vi "m2aadtView.vi"   [LabVIEW 2013, in "M2AADTViews.lvlib"]
uses:
  M2AADTViews.lvlib
  CommandFactory/CommandFactory.lvclass
  UserEvents/UserEvents.lvclass
  UserEvents/UserEvents.lvclass/UserEvents.ctl
  Typedefs/CommandSelector.ctl
  Typedefs/StateSelector.ctl
  Typedefs/M2AADTTypedefs.lvlib
  Controller/Controller.lvclass
  ConfigurationThisComponent/ConfigurationThisComponent.lvclass
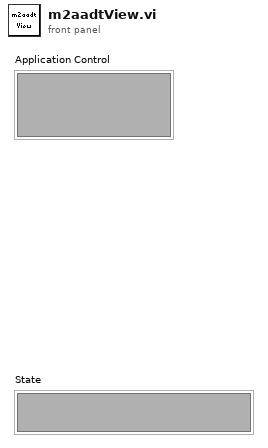
[diagram p1: front panel]
types:
  T1 = enum32{"invalid app kind", "Development System", "Run Time System", "Student Edition", "Embedded LabVIEW", "Evaluation", "Custom"}
  T2 = typedef "M2AADTTypedefs.lvlib/PubDataEvents.ctl" = cluster{"State":refnum<user-event>, "ErrorCode":refnum<user-event>, "OutputData":refnum<user-event>, "InputData":refnum<user-event>, "ControllerData":refnum<user-event>, "TestStatus":refnum<user-event>, "LogPath":refnum<user-event>, "StiffnessData":refnum<user-event>}
  T3 = typedef "M2AADTTypedefs.lvlib/SubDataEvents.ctl" = cluster{"Command":refnum<user-event>}
  T4 = cluster{"Event Registration Refnum":refnum<event-registration>, "Event Registration Refnum":refnum<event-registration>}
  T5 = typedef "M2AADTTypedefs.lvlib/CommandSelector.ctl" = enum16{"ClearError", "EnableMotion", "Exit", "ForceDemand", "StandBy", "Start", "StartAutomatedTest", "StopAutomatedTest", "StopMotion", "Update"}
  T6 = typedef "M2AADTTypedefs.lvlib/StateSelector.ctl" = enum16{"EndingCycleState", "FaultState", "InteractiveMotionState", "MovingToNewForceState", "OffState", "PausingState", "StandbyState", "StoppedState"}
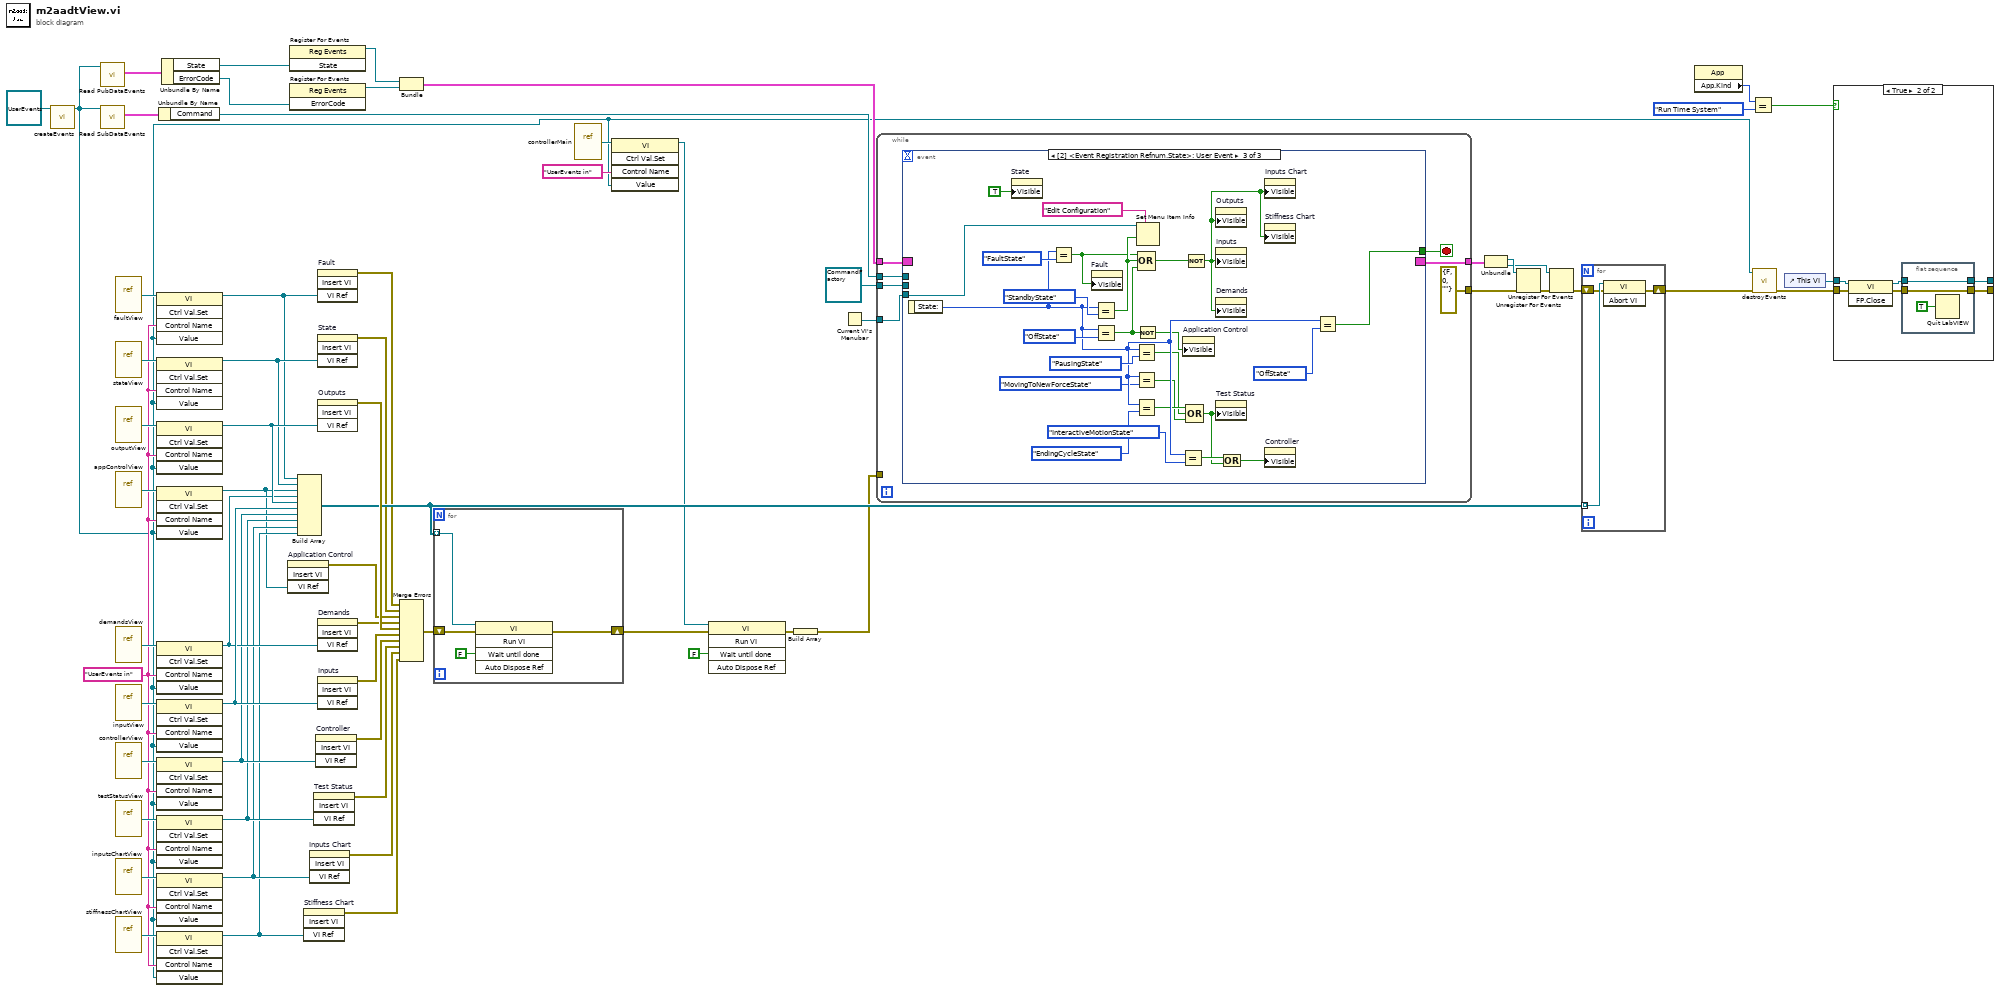
[diagram p0: block diagram]
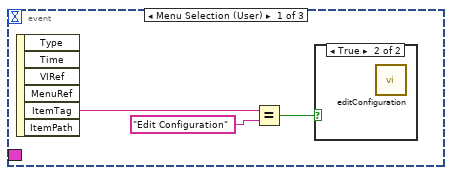
[diagram p3: hidden frame]
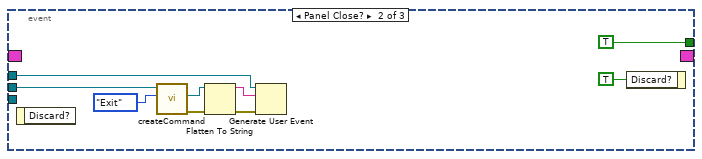
[diagram p5: hidden frame]
diagram:
  w6 = "UserEvents in" ("Control Name")
  n1 = call "createEvents.vi"("UserEvents in"=refnum<class "UserEvents.lvclass"> refnum) -> ("UserEvents out"=w5:refnum<class "UserEvents.lvclass">)  [unwired: 9 in, 1 out]
  n2 = call "Read PubDataEvents.vi"("UserEvents in"=w5) -> ("PubDataEvents"=w55:T2)  [unwired: 9 in, 1 out]
  n3 = call "Read SubDataEvents.vi"("UserEvents in"=w5) -> ("SubDataEvents"=w53:T3)  [unwired: 9 in, 1 out]
  n4 = vi-ref "faultView.vi"() -> (w7:refnum<vi>)
  n5 = vi-ref "stateView.vi"() -> (w10:refnum<vi>)
  n6 = vi-ref "outputView.vi"() -> (w35:refnum<vi>)
  n7 = vi-ref "appControlView.vi"() -> (w14:refnum<vi>)
  n8 = vi-ref "demandsView.vi"() -> (w29:refnum<vi>)
  n9 = vi-ref "inputView.vi"() -> (w43:refnum<vi>)
  n10 = vi-ref "controllerView.vi"() -> (w26:refnum<vi>)
  n11 = vi-ref "testStatusView.vi"() -> (w25:refnum<vi>)
  n12 = vi-ref "inputsChartView.vi"() -> (w20:refnum<vi>)
  n13 = vi-ref "stiffnessChartView.vi"() -> (w17:refnum<vi>)
  n14 = invoke class="VI" method="Ctrl Val.Set"(reference=w7, "Control Name"=w6, "Value"=w5) -> (reference out=w4:refnum<vi>)  [unwired: 2 in, 4 out]
  n15 = invoke class="VI" method="Ctrl Val.Set"(reference=w10, "Control Name"=w6, "Value"=w5) -> (reference out=w9:refnum<vi>)  [unwired: 2 in, 4 out]
  n16 = invoke class="VI" method="Ctrl Val.Set"(reference=w35, "Control Name"=w6, "Value"=w5) -> (reference out=w34:refnum<vi>)  [unwired: 2 in, 4 out]
  n17 = invoke class="VI" method="Ctrl Val.Set"(reference=w14, "Control Name"=w6, "Value"=w5) -> (reference out=w12:refnum<vi>)  [unwired: 2 in, 4 out]
  n18 = invoke class="VI" method="Ctrl Val.Set"(reference=w29, "Control Name"=w6, "Value"=w5) -> (reference out=w28:refnum<vi>)  [unwired: 2 in, 4 out]
  n19 = invoke class="VI" method="Ctrl Val.Set"(reference=w43, "Control Name"=w6, "Value"=w5) -> (reference out=w33:refnum<vi>)  [unwired: 2 in, 4 out]
  n20 = invoke class="VI" method="Ctrl Val.Set"(reference=w26, "Control Name"=w6, "Value"=w5) -> (reference out=w24:refnum<vi>)  [unwired: 2 in, 4 out]
  n21 = invoke class="VI" method="Ctrl Val.Set"(reference=w25, "Control Name"=w6, "Value"=w5) -> (reference out=w23:refnum<vi>)  [unwired: 2 in, 4 out]
  n22 = invoke class="VI" method="Ctrl Val.Set"(reference=w20, "Control Name"=w6, "Value"=w5) -> (reference out=w18:refnum<vi>)  [unwired: 2 in, 4 out]
  n23 = invoke class="VI" method="Ctrl Val.Set"(reference=w17, "Control Name"=w6, "Value"=w5) -> (reference out=w16:refnum<vi>)  [unwired: 2 in, 4 out]
  n24 = Unbundle By Name(w53) -> ("Command"=w52:refnum<user-event>)
  n25 = Unbundle By Name(w55) -> ("State"=w51:refnum<user-event>, "ErrorCode"=w49:refnum<user-event>)
  n26 = invoke on="Application Control" class="SubPnl" method="Insert VI"("VI Ref"=w12) -> (error out=w13:errorcluster)  [unwired: 3 in, 3 out]
  n27 = register-events(w51) -> (reference out=w50:refnum<event-registration>)  [unwired: 2 in, 1 out]
  n28 = register-events(w49) -> (reference out=w48:refnum<event-registration>)  [unwired: 2 in, 1 out]
  n29 = Build Array(w4, w9, w12, w28, w34, w33, w24, w23, w18, w16) -> (w58:refnum<vi>[])
  n30 = invoke on="Stiffness Chart" class="SubPnl" method="Insert VI"("VI Ref"=w16) -> (error out=w15:errorcluster)  [unwired: 3 in, 3 out]
  n31 = invoke on="Inputs Chart" class="SubPnl" method="Insert VI"("VI Ref"=w18) -> (error out=w19:errorcluster)  [unwired: 3 in, 3 out]
  n32 = invoke on="Test Status" class="SubPnl" method="Insert VI"("VI Ref"=w23) -> (error out=w21:errorcluster)  [unwired: 3 in, 3 out]
  n33 = invoke on="Controller" class="SubPnl" method="Insert VI"("VI Ref"=w24) -> (error out=w22:errorcluster)  [unwired: 3 in, 3 out]
  n34 = invoke on="Fault" class="SubPnl" method="Insert VI"("VI Ref"=w4) -> (error out=w3:errorcluster)  [unwired: 3 in, 3 out]
  n35 = invoke on="State" class="SubPnl" method="Insert VI"("VI Ref"=w9) -> (error out=w8:errorcluster)  [unwired: 3 in, 3 out]
  n36 = invoke on="Outputs" class="SubPanel" method="Insert VI"("VI Ref"=w34) -> (error out=w61:errorcluster)  [unwired: 3 in, 3 out]
  n37 = invoke on="Demands" class="SubPanel" method="Insert VI"("VI Ref"=w28) -> (error out=w27:errorcluster)  [unwired: 3 in, 3 out]
  n38 = invoke on="Inputs" class="SubPnl" method="Insert VI"("VI Ref"=w33) -> (error out=w60:errorcluster)  [unwired: 3 in, 3 out]
  n39 = Bundle("Event Registration Refnum"=w50, "Event Registration Refnum"=w48) -> (w41:T4)  [unwired: 1 in]
  n40 = Merge Errors(w3, w8, w13, w27, w61, w60, w22, w21, w19, w15) -> (w59:errorcluster)
  n41 = for {
    tunnel: w58 -> [w68] mode=indexing
    shift-right: [w67] -> w11
    shift-left: w59 -> [w66]
    n42 = invoke class="VI" method="Run VI"(reference=w68, error in=w66, "Wait until done"=FALSE ("Wait Until Done")) -> (error out=w67:errorcluster)  [unwired: 2 in, 4 out]
  }
  n43 = vi-ref "controllerMain.vi"() -> (w46:refnum<vi>)
  n44 = invoke class="VI" method="Ctrl Val.Set"(reference=w46, "Control Name"="UserEvents in", "Value"=w5) -> (reference out=w44:refnum<vi>)  [unwired: 2 in, 4 out]
  n45 = invoke class="VI" method="Run VI"(reference=w44, error in=w11, "Wait until done"=FALSE ("Wait Until Done")) -> (error out=w30:errorcluster)  [unwired: 2 in, 4 out]
  n46 = Build Array(w30) -> (w31:errorcluster[])
  n47 = Current VI's Menubar() -> (w56:refnum<k9>)
  n48 = while {
    tunnel: refnum<class "CommandFactory.lvclass"> refnum ("CommandFactory.lvclass") -> [w72]
    tunnel: [errorcluster {"status"=FALSE, "code"=0, "source"=""} ("error out")] -> w42
    tunnel: w56 -> [w70]
    tunnel: w41 -> [w74]
    tunnel: w52 -> [w71]
    tunnel: [w69] -> w40
    tunnel: w31 -> [_]
    stop <- w73 stop-if-true
    n49 = event shown="[2] <Event Registration Refnum.State>: User Event" {
      selector: w74 -> [_ _ _]
      dyn-events: [_ _ _] -> w69
      timeout: _ -> [_ _ _]
      tunnel: [_ TRUE w106] -> w73
      tunnel: w72 -> [_ w82 _]
      tunnel: w71 -> [_ w79 _]
      tunnel: w70 -> [_ _ w108]
      event Menu Selection (User) {
        n50 = event-data() -> ("ItemTag"=w76:string)  [unwired: 1 in, 5 out]
        n51 = Equal?(x=w76, y="Edit Configuration") -> (x = y?=w78:bool)
        n52 = case shown="True" w78 {
          frame False {
          }
          frame True {
            n53 = call "editConfiguration.vi"() -> ()  [unwired: 10 in, 2 out]
          }
        }
      }
      event Panel Close? {
        n54 = event-data() -> ()  [unwired: 1 in, 1 out]
        n55 = call-dynamic "createCommand.vi"("Command"=CommandSelector."Exit", "CommandFactory in"=w82) -> ("error out"=w87:errorcluster, "command"=w86:refnum<class "Command.lvclass">)  [unwired: 7 in, 1 out]
        n56 = Flatten To String(anything=w86, error in (no error)=w87) -> (data string=w80:string, error out=w81:errorcluster)  [unwired: 2 in, 1 out]
        n57 = Generate User Event(user event=w79, event data cluster=w80, error in=w81) -> ()  [unwired: 1 in, 2 out]
        n58 = event-data("Discard?"=TRUE) -> ()  [unwired: 1 in, 1 out]
      }
      event User Event {
        n59 = event-data() -> ("State:"=w101:T6)  [unwired: 1 in]
        n60 = property on="State" class="SubPnl"("Visible"=TRUE) -> ()  [unwired: 2 in, 2 out]
        n61 = Equal?(x=w101, y=StateSelector."FaultState") -> (x = y?=w88:bool)
        n62 = property on="Fault" class="SubPnl"("Visible"=w88) -> ()  [unwired: 2 in, 2 out]
        n63 = Equal?(x=w101, y=StateSelector."StandbyState") -> (x = y?=w105:bool)
        n64 = Equal?(x=w101, y=StateSelector."OffState") -> (x = y?=w90:bool)
        n65 = Equal?(x=w101, y=StateSelector."PausingState") -> (x = y?=w98:bool)
        n66 = Equal?(x=w101, y=StateSelector."MovingToNewForceState") -> (x = y?=w97:bool)
        n67 = Equal?(x=w101, y=StateSelector."EndingCycleState") -> (x = y?=w99:bool)
        n68 = Not(x=w90) -> (.not. x?=w91:bool)
        n69 = Set Menu Item Info(7:"Edit Configuration" ("item name"), 9:w105, 11:w108) -> ()  [unwired: 4 in, 2 out]
        n70 = Compound Arithmetic op=OR(w88, w105, w90) -> (w104:bool)
        n71 = Equal?(x=w101, y=StateSelector."InteractiveMotionState") -> (x = y?=w96:bool)
        n72 = property on="Application Control" class="SubPnl"("Visible"=w91) -> ()  [unwired: 2 in, 2 out]
        n73 = Not(x=w104) -> (.not. x?=w92:bool)
        n74 = Compound Arithmetic op=OR(w99, w98, w97) -> (w93:bool)
        n75 = property on="Outputs" class="SubPnl"("Visible"=w92) -> ()  [unwired: 2 in, 2 out]
        n76 = property on="Inputs" class="SubPnl"("Visible"=w92) -> ()  [unwired: 2 in, 2 out]
        n77 = property on="Demands" class="SubPnl"("Visible"=w92) -> ()  [unwired: 2 in, 2 out]
        n78 = property on="Test Status" class="SubPnl"("Visible"=w93) -> ()  [unwired: 2 in, 2 out]
        n79 = Compound Arithmetic op=OR(w96, w93) -> (w95:bool)
        n80 = property on="Inputs Chart" class="SubPnl"("Visible"=w92) -> ()  [unwired: 2 in, 2 out]
        n81 = property on="Stiffness Chart" class="SubPnl"("Visible"=w92) -> ()  [unwired: 2 in, 2 out]
        n82 = property on="Controller" class="SubPnl"("Visible"=w95) -> ()  [unwired: 2 in, 2 out]
        n83 = Equal?(x=w101, y=StateSelector."OffState") -> (x = y?=w106:bool)
      }
    }
  }
  n84 = Unbundle(w40) -> ("Event Registration Refnum"=w39:refnum<event-registration>, "Event Registration Refnum"=w37:refnum<event-registration>)
  n85 = Unregister For Events(event registration refnum=w39, error in=w42) -> (error out=w38:errorcluster)
  n86 = Unregister For Events(event registration refnum=w37, error in=w38) -> (error out=w36:errorcluster)
  n87 = for {
    tunnel: w58 -> [w115] mode=indexing
    shift-right: [w113] -> w32
    shift-left: w36 -> [w114]
    n88 = invoke class="VI" method="Abort VI"(reference=w115, error in=w114) -> (error out=w113:errorcluster)  [unwired: 1 in, 2 out]
  }
  n89 = property class="App"() -> ("App.Kind"=w64:T1)  [unwired: 2 in, 2 out]
  n90 = Equal?(x=w64, y=T1."Run Time System") -> (x = y?=w62:bool)
  n91 = call "destroyEvents.vi"("error in (no error)"=w32, "UserEvents in"=w5) -> ("error out"=w1:errorcluster)  [unwired: 8 in, 1 out]
  n92 = control-ref of="This VI"() -> (w2:refnum<vi>)
  n93 = case shown="True" w62 {
    tunnel: w2 -> [w117 w123]
    tunnel: w1 -> [w116 w122]
    tunnel: [w117 w120] -> _
    tunnel: [w116 w118] -> _
    frame False {
    }
    frame True {
      n94 = invoke class="VI" method="FP.Close"(reference=w123, error in=w122) -> (reference out=w119:refnum<vi>, error out=w121:errorcluster)  [unwired: 1 in, 1 out]
      n95 = flat-sequence {
        tunnel: w121 -> [w124]
        tunnel: [w125] -> w120
        tunnel: w119 -> [w125]
        tunnel: [w124] -> w118
        frame #0 {
          n96 = Quit LabVIEW(quit? (T)=TRUE) -> ()
        }
      }
    }
  }
